vi "2D_rand.vi"(10 "column_number":i32, 11 "row_number":i32) -> (3 "2D_Rand":dbl[][](array[numeric]))   [LabVIEW 2014]
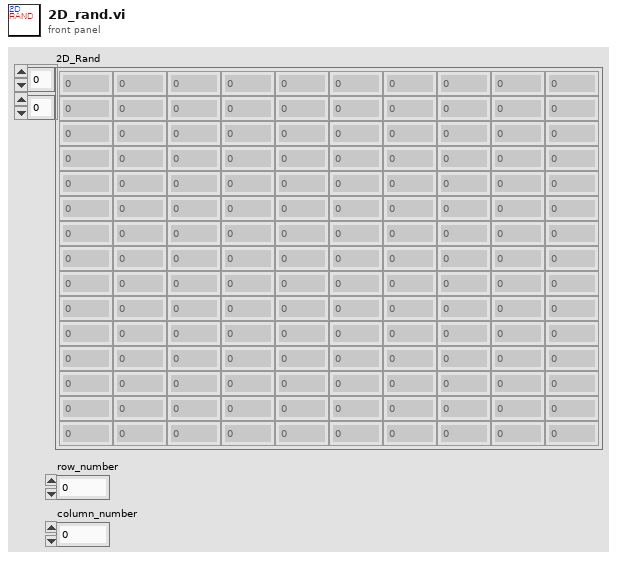
[diagram p1: front panel]
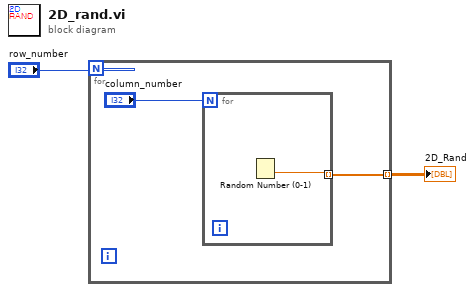
[diagram p0: block diagram]
diagram:
  n1 = for {
    N: "row_number" -> [_]
    tunnel: [w4] -> w2 mode=indexing
    n2 = for {
      N: "column_number" -> [_]
      tunnel: [w5] -> w4 mode=indexing
      n3 = Random Number (0-1)() -> (number: 0 to 1=w5:dbl)
    }
  }
  "2D_Rand" <- w2
